vi "Fundamentals.vi"() -> ()   [LabVIEW 2013]
uses:
  LapDog.Messaging/MessageQueue/MessageQueue.lvclass
  LapDog.Messaging/Message/Message.lvclass
  LapDog.Messaging/ErrorMsg/ErrorMsg.lvclass
  LapDog.Messaging/MessageQueue/EnqueueMessage(MsgObj).vi
  LapDog.Messaging/MessageQueue/EnqueueMessage(MsgName).vi
  LapDog.Messaging.NativeTypes/I32Msg/I32Msg.lvclass
panel:
  out "InLmt":bool caption="Within Limits?"
  in  "LowLmt":i32=-2 caption="Lower Limit"
  in  "UpLmt":i32=2 caption="Upper Limit"
  out "CurVal":i32 caption="Current Value"
  in  "DecBtn":bool
  in  "IncBtn":bool
  in  "MsgName":string caption="Message Name"
  in  "SendBtn":bool
  in  "GenError":bool
  # "This example illustrates the basic principles of the LapDog.Messaging library (LML).  The front panel is used only to generate messages for the Message Handler and observe the resultant behavior.  It is not intended to be a proper application user interface.\n\nThe Application Messages group creates and sends messages relating to the application's business purpose.  The Framework Messages group is used to observe the framework's built in response to common situations.\n\nPressing the Simulate Error button causes an error cluster to be sent to the DequeueMessage's error in terminal, simulating an unhandled error in the previous message's error handling case.  LML responds to this input error by returning a QueueErrorIn ErrorObj message.\n\nThe Send Arb Msg button sends a message with the name defined in the Message Name text box.  Any messages with names not explicitly handled by the message handler are handled by the Default message handler.  Note that messages without a name return the name of the message's class rather than an empty string.\n\nTurn on execution highlighting and explore how this message handler loop reacts to the following messages sent using the Send Arb Msg button:\n\"Increment\"\n\"LowerLimitChanged\"\n\"SimulatedError\""
  # "Application Messages"
  # "Framework Messages"
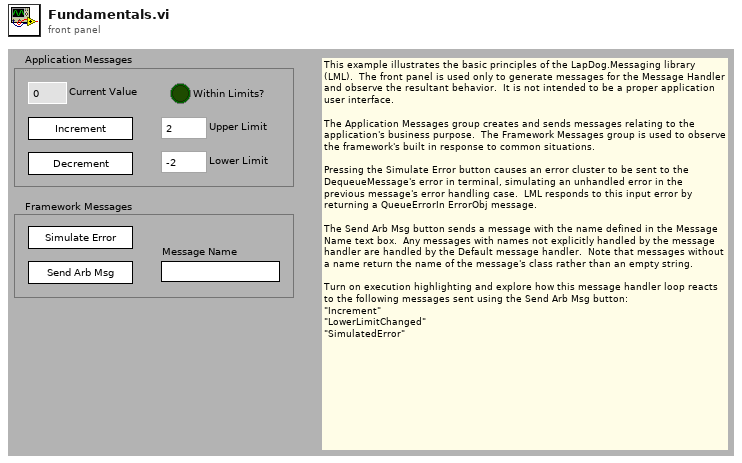
[diagram p1: front panel]
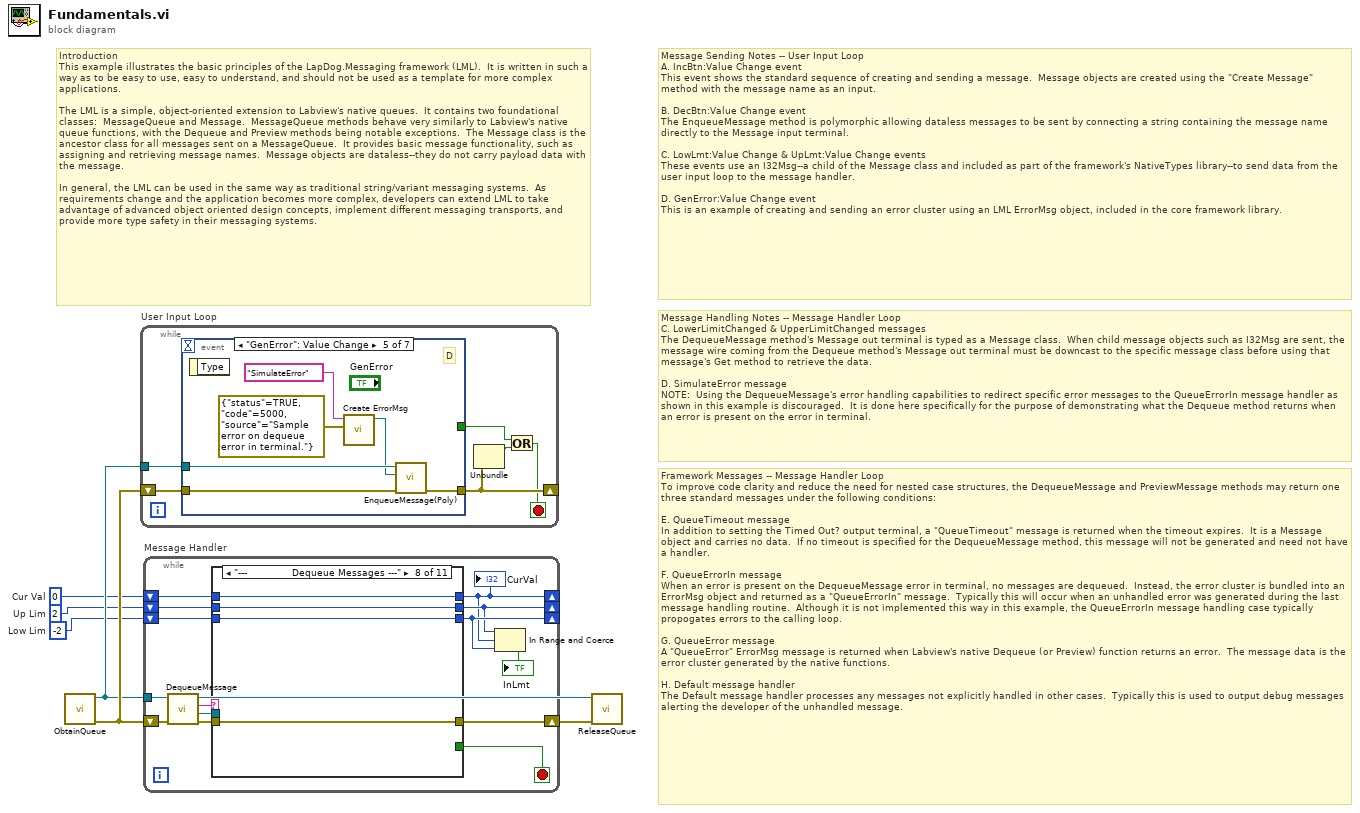
[diagram p0: block diagram]
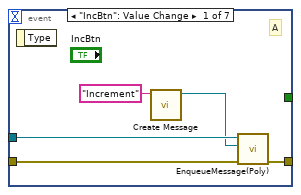
[diagram p2: hidden frame]
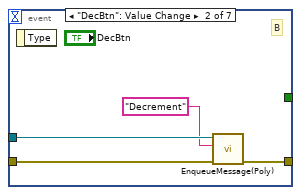
[diagram p3: hidden frame]
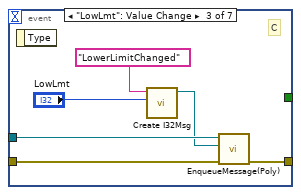
[diagram p4: hidden frame]
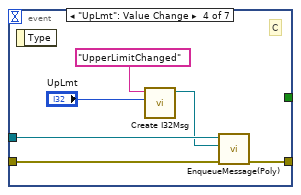
[diagram p5: hidden frame]
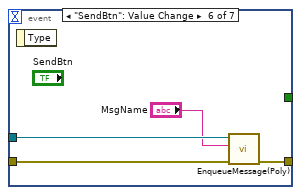
[diagram p6: hidden frame]
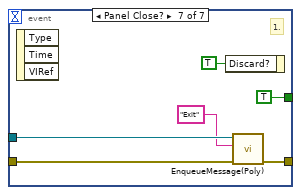
[diagram p7: hidden frame]
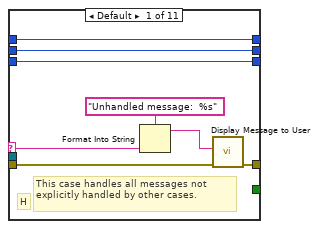
[diagram p8: hidden frame]
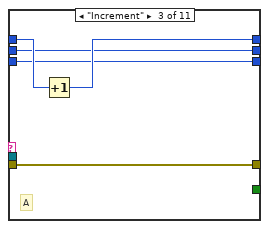
[diagram p10: hidden frame]
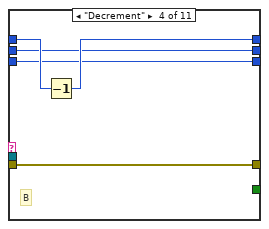
[diagram p11: hidden frame]
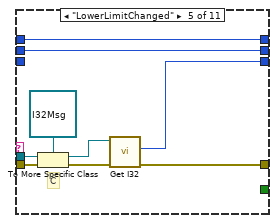
[diagram p12: hidden frame]
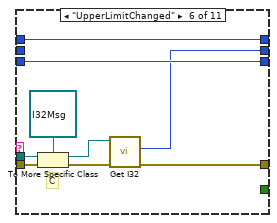
[diagram p13: hidden frame]
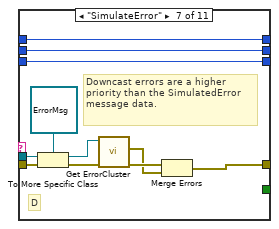
[diagram p14: hidden frame]
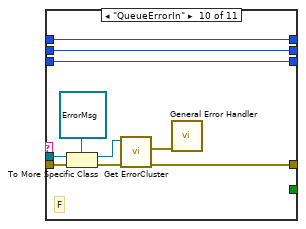
[diagram p16: hidden frame]
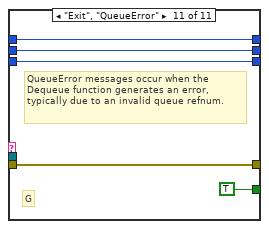
[diagram p17: hidden frame]
diagram:
  w1 = -2  # Low Lim
  w2 = 2  # Up Lim
  w3 = 0  # Cur Val
  # "Framework Messages -- Message Handler Loop\nTo improve code clarity and reduce the need for nested case structures, the DequeueMessage and PreviewMessage methods may return one three standard messages under the following conditions:\n\nE. QueueTimeout message\nIn addition to setting the Timed Out? output terminal, a \"QueueTimeout\" message is returned when the timeout expires.  It is a Message object and carries no data.  If no timeout is specified for the DequeueMessage method, this message will not be generated and need not have a handler.\n\nF. QueueErrorIn message\nWhen an error is present on the DequeueMessage error in terminal, no messages are dequeued.  Instead, the error cluster is bundled into an ErrorMsg object and returned as a \"QueueErrorIn\" message.  Typically this will occur when an unhandled error was generated during the last message handling routine.  Although it is not implemented this way in this example, the QueueErrorIn message handling case typically propogates errors to the calling loop.\n\nG. QueueError message\nA \"QueueError\" ErrorMsg message is returned when Labview's native Dequeue (or Preview) function returns an error.  The message data is the error cluster generated by the native functions.\n\nH. Default message handler\nThe Default message handler processes any messages not explicitly handled in other cases.  Typically this is used to output debug messages alerting the developer of the unhandled message."
  # "Message Handling Notes -- Message Handler Loop\nC. LowerLimitChanged & UpperLimitChanged messages\nThe DequeueMessage method's Message out terminal is typed as a Message class.  When child message objects such as I32Msg are sent, the message wire coming from the Dequeue method's Message out terminal must be downcast to the specific message class before using that message's Get method to retrieve the data.\n\nD. SimulateError message\nNOTE:  Using the DequeueMessage's error handling capabilities to redirect specific error messages to the QueueErrorIn message handler as shown in this example is discouraged.  It is done here specifically for the purpose of demonstrating what the Dequeue method returns when an error is present on the error in terminal."
  # "Introduction\nThis example illustrates the basic principles of the LapDog.Messaging framework (LML).  It is written in such a way as to be easy to use, easy to understand, and should not be used as a template for more complex applications.\n\nThe LML is a simple, object-oriented extension to Labview's native queues.  It contains two foundational classes:  MessageQueue and Message.  MessageQueue methods behave very similarly to Labview's native queue functions, with the Dequeue and Preview methods being notable exceptions.  The Message class is the ancestor class for all messages sent on a MessageQueue.  It provides basic message functionality, such as assigning and retrieving message names.  Message objects are dataless--they do not carry payload data with the message.\n\nIn general, the LML can be used in the same way as traditional string/variant messaging systems.  As requirements change and the application becomes more complex, developers can extend LML to take advantage of advanced object oriented design concepts, implement different messaging transports, and provide more type safety in their messaging systems."
  # "Message Sending Notes -- User Input Loop\nA. IncBtn:Value Change event \nThis event shows the standard sequence of creating and sending a message.  Message objects are created using the \"Create Message\" method with the message name as an input.\n\nB. DecBtn:Value Change event \nThe EnqueueMessage method is polymorphic allowing dataless messages to be sent by connecting a string containing the message name directly to the Message input terminal.\n\nC. LowLmt:Value Change & UpLmt:Value Change events\nThese events use an I32Msg--a child of the Message class and included as part of the framework's NativeTypes library--to send data from the user input loop to the message handler.\n\nD. GenError:Value Change event\nThis is an example of creating and sending an error cluster using an LML ErrorMsg object, included in the core framework library."
  n1 = call "ObtainQueue.vi"() -> ("error out"=w6:errorcluster, "MessageQueue out"=w4:refnum<class "MessageQueue.lvclass">)  [unwired: 9 in, 1 out]
  n2 = while "User Input Loop" {
    tunnel: w4 -> [w11]
    shift-right: [w10] -> _
    shift-left: w6 -> [w12]
    stop <- w8 stop-if-true
    n3 = event shown="[4] \"GenError\": Value Change" {
      selector: _ -> [_ _ _ _ _ _ _]
      dyn-events: _ -> [_ _ _ _ _ _ _]
      timeout: _ -> [_ _ _ _ _ _ _]
      tunnel: [w16 w20 w26 w32 w38 w42 w48] -> w10
      tunnel: w12 -> [w17 w21 w27 w33 w39 w43 w47]
      tunnel: w11 -> [w15 w19 w25 w31 w37 w41 w46]
      tunnel: [_ _ _ _ _ _ TRUE] -> w7
      event "IncBtn": Value Change {
        # "A"
        n4 = event-data() -> ()  [unwired: 1 in, 1 out]
        n5 = call "Create Message.vi"("Message Name"="Increment") -> ("Message out"=w13:refnum<class "Message.lvclass">)  [unwired: 9 in, 1 out]
        n6 = call-poly "EnqueueMessage(Poly).vi"("error in (no error)"=w17, "Message"=w13, "MessageQueue in"=w15) -> ("error out"=w16:errorcluster)  [unwired: 6 in, 2 out]
      }
      event "DecBtn": Value Change {
        # "B"
        n7 = event-data() -> ()  [unwired: 1 in, 1 out]
        n8 = call-poly "EnqueueMessage(Poly).vi"("error in (no error)"=w21, "Message Name"="Decrement", "MessageQueue in"=w19) -> ("error out"=w20:errorcluster)  [unwired: 6 in, 2 out]
      }
      event "LowLmt": Value Change {
        # "C"
        n9 = event-data() -> ()  [unwired: 1 in, 1 out]
        n10 = call "Create I32Msg.vi"("Message Data"="LowLmt", "Message Name"="LowerLimitChanged") -> ("I32Msg out"=w22:refnum<class "I32Msg.lvclass">)  [unwired: 8 in, 1 out]
        n11 = call-poly "EnqueueMessage(Poly).vi"("error in (no error)"=w27, "Message"=w22, "MessageQueue in"=w25) -> ("error out"=w26:errorcluster)  [unwired: 6 in, 2 out]
      }
      event "UpLmt": Value Change {
        # "C"
        n12 = event-data() -> ()  [unwired: 1 in, 1 out]
        n13 = call "Create I32Msg.vi"("Message Data"="UpLmt", "Message Name"="UpperLimitChanged") -> ("I32Msg out"=w28:refnum<class "I32Msg.lvclass">)  [unwired: 8 in, 1 out]
        n14 = call-poly "EnqueueMessage(Poly).vi"("error in (no error)"=w33, "Message"=w28, "MessageQueue in"=w31) -> ("error out"=w32:errorcluster)  [unwired: 6 in, 2 out]
      }
      event "GenError": Value Change {
        # "D"
        n15 = event-data() -> ()  [unwired: 1 in, 1 out]
        n16 = call "Create ErrorMsg.vi"("Error Cluster"=errorcluster {"status"=TRUE, "code"=5000, "source"="Sample error on dequeue error in terminal."} ("error out"), "Message Name"="SimulateError") -> ("ErrorMsg out"=w36:refnum<class "ErrorMsg.lvclass">)  [unwired: 8 in, 1 out]
        n17 = call-poly "EnqueueMessage(Poly).vi"("error in (no error)"=w39, "Message"=w36, "MessageQueue in"=w37) -> ("error out"=w38:errorcluster)  [unwired: 6 in, 2 out]
      }
      event "SendBtn": Value Change {
        n18 = event-data() -> ()  [unwired: 1 in, 1 out]
        n19 = call-poly "EnqueueMessage(Poly).vi"("error in (no error)"=w43, "Message Name"="MsgName", "MessageQueue in"=w41) -> ("error out"=w42:errorcluster)  [unwired: 6 in, 2 out]
      }
      event Panel Close? {
        # "1."
        n20 = event-data() -> ()  [unwired: 1 in, 3 out]
        n21 = event-data("Discard?"=TRUE) -> ()  [unwired: 1 in, 1 out]
        n22 = call-poly "EnqueueMessage(Poly).vi"("error in (no error)"=w47, "Message Name"="Exit", "MessageQueue in"=w46) -> ("error out"=w48:errorcluster)  [unwired: 6 in, 2 out]
      }
    }
    n23 = Unbundle(w10) -> ("status"=w9:bool)  [unwired: 2 out]
    n24 = Or(x=w7, y=w9) -> (x .or. y?=w8:bool)
  }
  n25 = while "Message Handler" {
    tunnel: w4 -> [w62]
    shift-right: [w58] -> w5
    shift-left: w6 -> [w63]
    shift-right: [w50] -> _
    shift-left: w3 -> [w57]
    shift-right: [w51] -> _
    shift-left: w2 -> [w56]
    shift-right: [w54] -> _
    shift-left: w1 -> [w55]
    stop <- w52 stop-if-true
    n26 = call-dynamic "DequeueMessage.vi"("error in (no error)"=w63, "MessageQueue in"=w62) -> ("error out"=w59:errorcluster, "Message out"=w60:refnum<class "Message.lvclass">, "Message Name"=w61:string)  [unwired: 5 in, 2 out]
    n27 = case shown="\"---               Dequeue Messages ---\"" w61 {
      selector: w61 -> [w66 _ _ _ _ _ _ _ _ _ _]
      tunnel: w60 -> [_ _ _ _ w91 w97 w110 _ _ w128 _]
      tunnel: w59 -> [w68 w72 w80 w85 w92 w98 w111 w115 w122 w129 w134]
      tunnel: [w67 w72 w80 w85 w88 w95 w104 w115 w122 w125 w134] -> w58
      tunnel: [w71 w75 w78 w83 w94 w103 w114 w118 w121 w132 w137] -> w50
      tunnel: w57 -> [w71 w75 w79 w84 w94 w103 w114 w118 w121 w132 w137]
      tunnel: w56 -> [w69 w74 w76 w82 w93 _ w113 w117 w119 w131 w136]
      tunnel: [w69 w74 w76 w82 w93 w96 w113 w117 w119 w131 w136] -> w51
      tunnel: w55 -> [w70 w73 w77 w81 _ w102 w112 w116 w120 w130 w135]
      tunnel: [w70 w73 w77 w81 w87 w102 w112 w116 w120 w130 w135] -> w54
      tunnel: [_ _ _ _ _ _ _ _ _ _ TRUE] -> w52
      frame Default {
        # "H"
        # "This case handles all messages not explicitly handled by other cases."
        n28 = Format Into String(format string="Unhandled message:  %s", w66) -> (resulting string=w65:string)  [unwired: 2 in, 1 out]
        n29 = call "Display Message to User"("error in (no error)"=w68, "Message"=w65) -> ("error out"=w67:errorcluster)  [unwired: 8 in, 1 out]
      }
      frame "---               Application Messages ---" {
      }
      frame "Increment" {
        # "A"
        n30 = Increment(x=w79) -> (x+1=w78:i32)
      }
      frame "Decrement" {
        # "B"
        n31 = Decrement(x=w84) -> (x-1=w83:i32)
      }
      frame "LowerLimitChanged" {
        # "C"
        n32 = To More Specific Class(target class=refnum<class "I32Msg.lvclass"> refnum ("I32Msg"), reference=w91, error in=w92) -> (specific class reference=w90:refnum<class "I32Msg.lvclass">, error out=w89:errorcluster)
        n33 = call-dynamic "Get I32.vi"("error in (no error)"=w89, "I32Msg in"=w90) -> ("error out"=w88:errorcluster, "Message Data"=w87:i32)  [unwired: 7 in, 1 out]
      }
      frame "UpperLimitChanged" {
        # "C"
        n34 = To More Specific Class(target class=refnum<class "I32Msg.lvclass"> refnum ("I32Msg"), reference=w97, error in=w98) -> (specific class reference=w101:refnum<class "I32Msg.lvclass">, error out=w100:errorcluster)
        n35 = call-dynamic "Get I32.vi"("error in (no error)"=w100, "I32Msg in"=w101) -> ("error out"=w95:errorcluster, "Message Data"=w96:i32)  [unwired: 7 in, 1 out]
      }
      frame "SimulateError" {
        # "Downcast errors are a higher priority than the SimulatedError message data."
        # "D"
        n36 = To More Specific Class(target class=refnum<class "ErrorMsg.lvclass"> refnum ("ErrorMsg in"), reference=w110, error in=w111) -> (specific class reference=w108:refnum<class "ErrorMsg.lvclass">, error out=w107:errorcluster)
        n37 = call-dynamic "Get ErrorCluster.vi"("error in (no error)"=w107, "ErrorMsg in"=w108) -> ("error out"=w106:errorcluster, "ErrorCluster"=w105:errorcluster)  [unwired: 7 in, 1 out]
        n38 = Merge Errors(w106, w105) -> (w104:errorcluster)
      }
      frame "---               Dequeue Messages ---" {
      }
      frame "QueueTimeout" {
        # "E"
        # "This standard message is sent when the dequeue prim times out.  (Dequeue timeouts are not used in this example.)"
      }
      frame "QueueErrorIn" {
        # "F"
        n39 = To More Specific Class(target class=refnum<class "ErrorMsg.lvclass"> refnum ("ErrorMsg"), reference=w128, error in=w129) -> (specific class reference=w124:refnum<class "ErrorMsg.lvclass">, error out=w126:errorcluster)
        n40 = call-dynamic "Get ErrorCluster.vi"("error in (no error)"=w126, "ErrorMsg in"=w124) -> ("error out"=w125:errorcluster, "ErrorCluster"=w123:errorcluster)  [unwired: 7 in, 1 out]
        n41 = call <vilib>:"General Error Handler.vi"("error in (no error)"=w123) -> ()  [unwired: 10 in, 5 out]
      }
      frame "Exit", "QueueError" {
        # "G"
        # "QueueError messages occur when the Dequeue function generates an error, typically due to an invalid queue refnum."
      }
    }
    "CurVal" <- w50
    n42 = In Range and Coerce(upper limit=w51, x=w50, lower limit=w54) -> (In Range?=→"InLmt":bool)  [unwired: 1 out]
  }
  n43 = call-dynamic "ReleaseQueue.vi"("error in (no error)"=w5, "MessageQueue in"=w4) -> ()  [unwired: 7 in, 3 out]
